vi "Read Child Attributes Map.vi"(11 "Actor in":refnum<class "Actor.lvclass">) -> (2 "Child Attributes Map":T1)   [LabVIEW 2020, in "jettl.lvlib" / "Actor.lvclass"]
uses:
  Actor.lvclass
  Child Actor Attributes Map.ctl
  jettl.lvlib
  Transport/Transport.lvclass
  Actor Attributes.ctl
  Msg/Msg.lvclass
  Msgs.ctl
  Msg Names.ctl
  Unified Layer.ctl
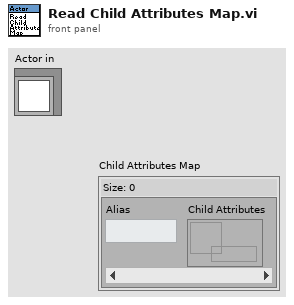
[diagram p1: front panel]
types:
  T1 = typedef "jettl.lvlib/Child Actor Attributes Map.ctl" = map{string, refnum<data-value>}
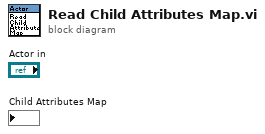
[diagram p0: block diagram]
diagram:
